vi "convert--chess_square (chess notation) to chessboard_index.vi"(1 "chess_square (chess notation)":T1) -> (0 "chessboard_index":T4)   [LabVIEW 2020, in "core.lvlib"]
uses:
  core.lvlib
  core_data/chessboard_index.ctl
  core_data/chess_square--chess notation.ctl
  core_data/file--enum.ctl
  core_data/rank--enum.ctl
  core_data/core_data.lvlib
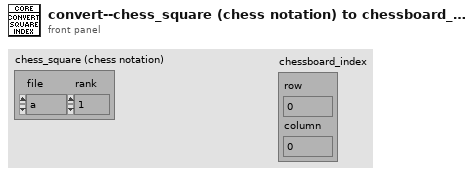
[diagram p1: front panel]
types:
  T1 = typedef "core.lvlib/core_data.lvlib/chess_square--chess notation.ctl" = cluster{"file":T2, "rank":T3}
  T2 = typedef "core.lvlib/core_data.lvlib/file--enum.ctl" = enum16{"a", "b", "c", "d", "e", "f", "g", "h"}
  T3 = typedef "core.lvlib/core_data.lvlib/rank--enum.ctl" = enum16{"1", "2", "3", "4", "5", "6", "7", "8"}
  T4 = typedef "core.lvlib/core_data.lvlib/chessboard_index.ctl" = cluster{"row":u8, "column":u8}
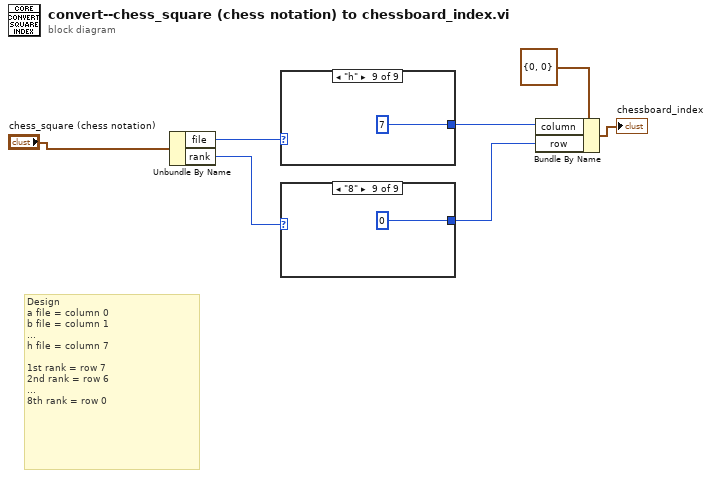
[diagram p0: block diagram]
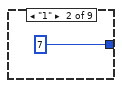
[diagram p3: hidden frame]
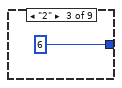
[diagram p4: hidden frame]
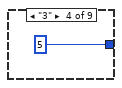
[diagram p5: hidden frame]
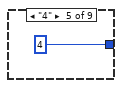
[diagram p6: hidden frame]
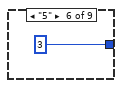
[diagram p7: hidden frame]
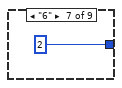
[diagram p8: hidden frame]
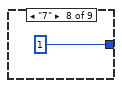
[diagram p9: hidden frame]
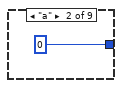
[diagram p11: hidden frame]
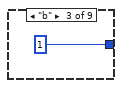
[diagram p12: hidden frame]
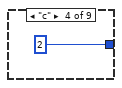
[diagram p13: hidden frame]
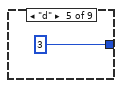
[diagram p14: hidden frame]
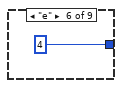
[diagram p15: hidden frame]
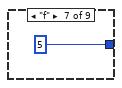
[diagram p16: hidden frame]
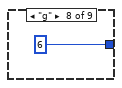
[diagram p17: hidden frame]
diagram:
  # "Design\na file = column 0\nb file = column 1\n...\nh file = column 7\n\n1st rank = row 7\n2nd rank = row 6\n...\n8th rank = row 0"
  n1 = Unbundle By Name("chess_square (chess notation)") -> ("file"=w6:T2, "rank"=w2:T3)
  n2 = case shown="\"h\"" w6 {
    tunnel: [_ u8 0 ("row") u8 1 ("row") u8 2 ("row") u8 3 ("row") u8 4 ("row") u8 5 ("row") u8 6 ("row") u8 7 ("row")] -> w3
    frame Default {
    }
    frame "a" {
    }
    frame "b" {
    }
    frame "c" {
    }
    frame "d" {
    }
    frame "e" {
    }
    frame "f" {
    }
    frame "g" {
    }
    frame "h" {
    }
  }
  n3 = case shown="\"8\"" w2 {
    tunnel: [_ u8 7 ("row") u8 6 ("row") u8 5 ("row") u8 4 ("row") u8 3 ("row") u8 2 ("row") u8 1 ("row") u8 0 ("row")] -> w1
    frame Default {
    }
    frame "1" {
    }
    frame "2" {
    }
    frame "3" {
    }
    frame "4" {
    }
    frame "5" {
    }
    frame "6" {
    }
    frame "7" {
    }
    frame "8" {
    }
  }
  n4 = Bundle By Name(cluster=T4 {"row"=0, "column"=0} ("chessboard_index"), "column"=w3, "row"=w1) -> (→"chessboard_index":T4)
